vi "PNG Chunk.vi"(10 "Data":string, 11 "Type":string) -> (3 "PNG Chunk":T1 {"CRC" format="%08x"})   [LabVIEW 2022 SP3, in "VI-Snippet.lvlib"]
doc: "Returns a PNG chunk cluster given the <b>Type</b> and <b>Data</b> strings."
uses:
  VI-Snippet.lvlib
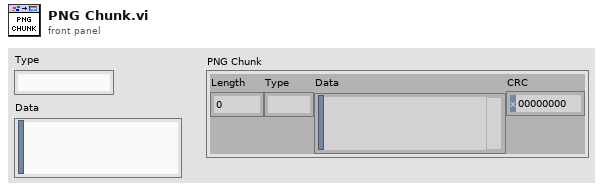
[diagram p1: front panel]
types:
  T1 = cluster{"Length":i32, "Type":string, "Data":string, "CRC":u32}
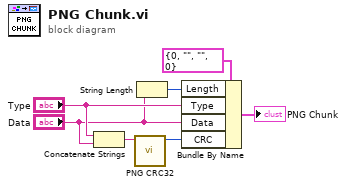
[diagram p0: block diagram]
diagram:
  n1 = Concatenate Strings("Type", "Data") -> (w2:string)
  n2 = call "PNG CRC32.vi"("String in"=w2) -> ("crc32 out"=w1:u32)  [unwired: 10 in]
  n3 = String Length(string="Data") -> (length=w5:i32)
  n4 = Bundle By Name(cluster=T1 {"Length"=0, "Type"="", "Data"="", "CRC"=0} ("Chunk"), "Length"=w5, "Type"="Type", "Data"="Data", "CRC"=w1) -> (→"PNG Chunk":T1)
